vi "XiXi-1(Divide I8[]).vi"(10 "X[-1]":i8[](array[numeric]), 11 "Xi":i8[][](array[numeric])) -> (2 "Remain":i8[][](array[numeric]), 3 "Yi":i8[][](array[numeric]))   [LabVIEW 2012]
doc: "Calculate sums of consecutive array elements. 0th element of output is equal to x(0)+ x(-1), where x(-1) is an optional scalar input that defaults to zero."
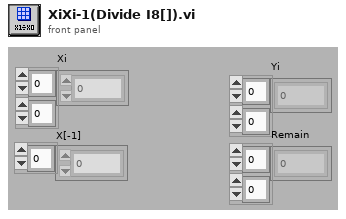
[diagram p1: front panel]
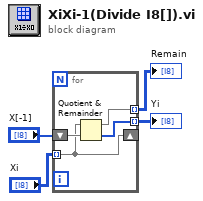
[diagram p0: block diagram]
diagram:
  n1 = for {
    shift-right: [w7] -> _
    shift-left: "X[-1]" -> [w8]
    tunnel: "Xi" -> [w7] mode=indexing
    tunnel: [w6] -> w2 mode=indexing
    tunnel: [w5] -> w1 mode=indexing
    n2 = Quotient & Remainder(x=w7, y=w8) -> (x-y*floor(x/y)=w5:i8[], floor(x/y)=w6:i8[])
  }
  "Yi" <- w2
  "Remain" <- w1
